vi "Get Number Vertical Speeds.vi"(11 "number":i32) -> (2 "function return":u32, 3 "number out":i32)   [LabVIEW 2018, in "Copy of Andor SDK.lvlib"]
doc: "EXPNETTYPE unsigned int WINAPI GetNumberVerticalSpeeds(int * number);"
uses:
  Copy of Andor SDK.lvlib
  <userlib>/Andor SDK/ATMCD32D.dll
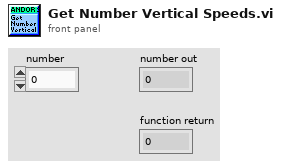
[diagram p1: front panel]
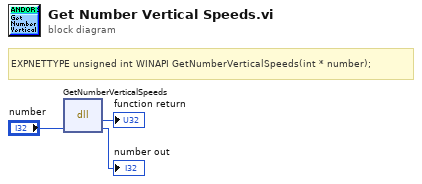
[diagram p0: block diagram]
diagram:
  # "EXPNETTYPE unsigned int WINAPI GetNumberVerticalSpeeds(int * number);"
  n1 = dll-call lib="C:/Program Files (x86)/National Instruments/LabVIEW 2018/user.lib/Andor SDK/ATMCD32D.*" fn="GetNumberVerticalSpeeds"("number"="number") -> (→"function return":u32, "number"=→"number out":i32)  [unwired: 3 in, 2 out]
